vi "fit function - LogMinusT.vi"(3 "output control":T1, 4 "data":T2, 5 "X":dbl[](array[numeric]), 6 "a":dbl[](array[numeric])) -> (0 "error out":errorcluster, 1 "f'(X,a)":dbl[][](array[numeric]), 2 "f(X,a)":dbl[](array[numeric]))   [LabVIEW 2015]
doc: "This template is the starting point for creating a model function to be passed to the Nonlinear Curve Fit.vi."
uses:
  <vilib>/gmath/NumericalOptimization/objective function data.ctl
  <vilib>/gmath/NumericalOptimization/LM_output select.ctl
  <vilib>/gmath/NI_Gmath.lvlib
panel:
  in  "fit":enum16{"other", "3par", "5par"}(ring)=enum."3par"
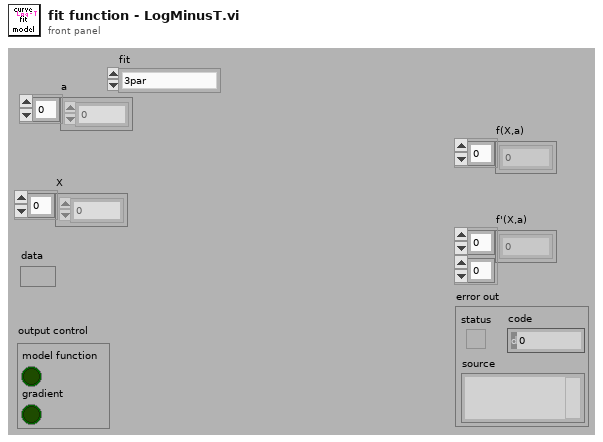
[diagram p1: front panel]
types:
  T1 = typedef "NI_Gmath.lvlib/LM_output select.ctl" = cluster{"model function":bool, "gradient":bool}
  T2 = typedef "NI_Gmath.lvlib/objective function data.ctl" = variant
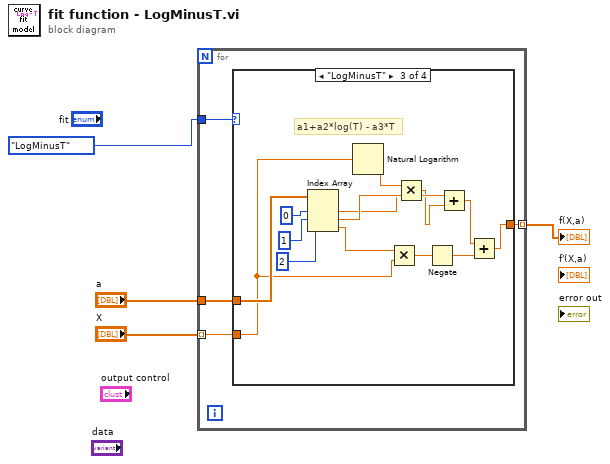
[diagram p0: block diagram]
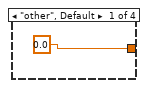
[diagram p2: hidden frame]
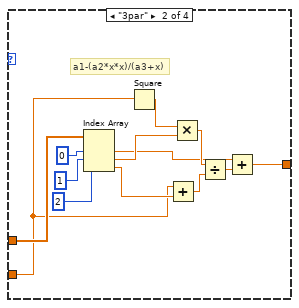
[diagram p3: hidden frame]
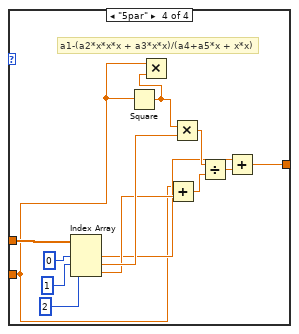
[diagram p4: hidden frame]
diagram:
  n1 = for {
    tunnel: "a" -> [w8]
    tunnel: "X" -> [w6] mode=indexing
    tunnel: [w7] -> w2 mode=indexing
    tunnel: enum16{"other", "3par", "5par", "LogMinusT"}."LogMinusT" ("action") -> [w5]
    n2 = case shown="\"LogMinusT\"" w5 {
      tunnel: w8 -> [_ w22 w36 w49]
      tunnel: [0.0 w12 w27 w39] -> w7
      tunnel: w6 -> [_ w11 w25 w38]
      frame "other", Default {
      }
      frame "3par" {
        # "a1-(a2*x*x)/(a3+x)"
        n3 = Index Array(array=w22, index #1=0 ("index"), index #2=1 ("index"), index #3=2 ("index")) -> (element #1=w14:dbl, element #2=w18:dbl, element #3=w17:dbl)
        n4 = Square(x=w11) -> (x^2=w10:dbl)
        n5 = Add(x=w11, y=w17) -> (x+y=w15:dbl)
        n6 = Multiply(x=w10, y=w18) -> (x*y=w16:dbl)
        n7 = Divide(x=w16, y=w15) -> (x/y=w13:dbl)
        n8 = Add(x=w14, y=w13) -> (x+y=w12:dbl)
      }
      frame "LogMinusT" {
        # "a1+a2*log(T) - a3*T"
        n9 = Index Array(array=w36, index #1=0 ("index"), index #2=1 ("index"), index #3=2 ("index")) -> (element #1=w31:dbl, element #2=w32:dbl, element #3=w26:dbl)
        n10 = Natural Logarithm(1:w25) -> (0:w30:dbl)
        n11 = Multiply(x=w26, y=w25) -> (x*y=w24:dbl)
        n12 = Multiply(x=w30, y=w32) -> (x*y=w29:dbl)
        n13 = Negate(x=w24) -> (-x=w23:dbl)
        n14 = Add(x=w31, y=w29) -> (x+y=w28:dbl)
        n15 = Add(x=w28, y=w23) -> (x+y=w27:dbl)
      }
      frame "5par" {
        # "a1-(a2*x*x*x + a3*x*x)/(a4+a5*x + x*x)"
        n16 = Index Array(array=w49, index #1=0 ("index"), index #2=1 ("index"), index #3=2 ("index")) -> (element #1=w41:dbl, element #2=w45:dbl, element #3=w44:dbl)
        n17 = Square(x=w38) -> (x^2=w37:dbl)
        n18 = Multiply(x=w38, y=w37) -> ()  [unwired: 1 out]
        n19 = Add(x=w38, y=w44) -> (x+y=w42:dbl)
        n20 = Multiply(x=w37, y=w45) -> (x*y=w43:dbl)
        n21 = Divide(x=w43, y=w42) -> (x/y=w40:dbl)
        n22 = Add(x=w41, y=w40) -> (x+y=w39:dbl)
      }
    }
  }
  "f(X,a)" <- w2
